vi "Globals.vi"(7 "action":T2, 8 "error in":errorcluster, 10 "Preliminary Settings":T1={"Nº of Scans (ns)"=3, "Pulse Frequency"=10000000.0} {"Pulse Frequency" min=1.0 format="%^#_6e"; "Nº of Scans (ns)" step=1}) -> (0 "error out":errorcluster, 2 "Preliminary Settings out":T1={"Nº of Scans (ns)"=3, "Pulse Frequency"=10000000.0} {"Pulse Frequency" min=1.0 format="%^#_6e"; "Nº of Scans (ns)" step=1})   [LabVIEW 2011]
uses:
  Globals.ctl
  Controls/Preliminary Settings.ctl
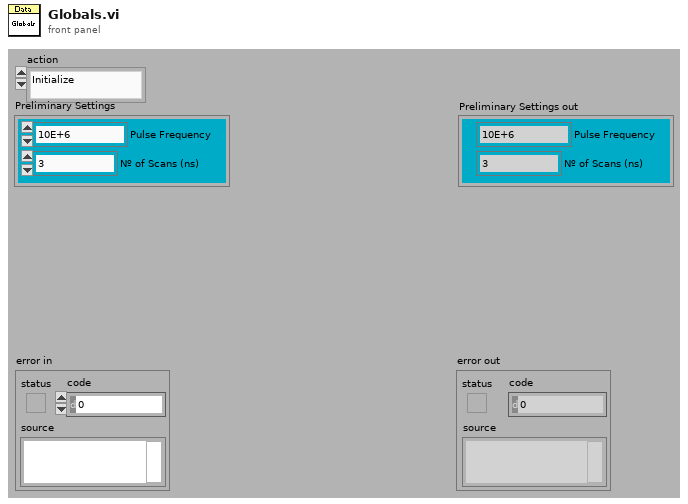
[diagram p1: front panel]
types:
  T1 = typedef "Preliminary Settings.ctl" = cluster{"Nº of Scans (ns)":u16, "Pulse Frequency":dbl}
  T2 = typedef "Globals.ctl" = enum16{"Initialize", "Set Preliminary Settings", "Get Preliminary Settings"}
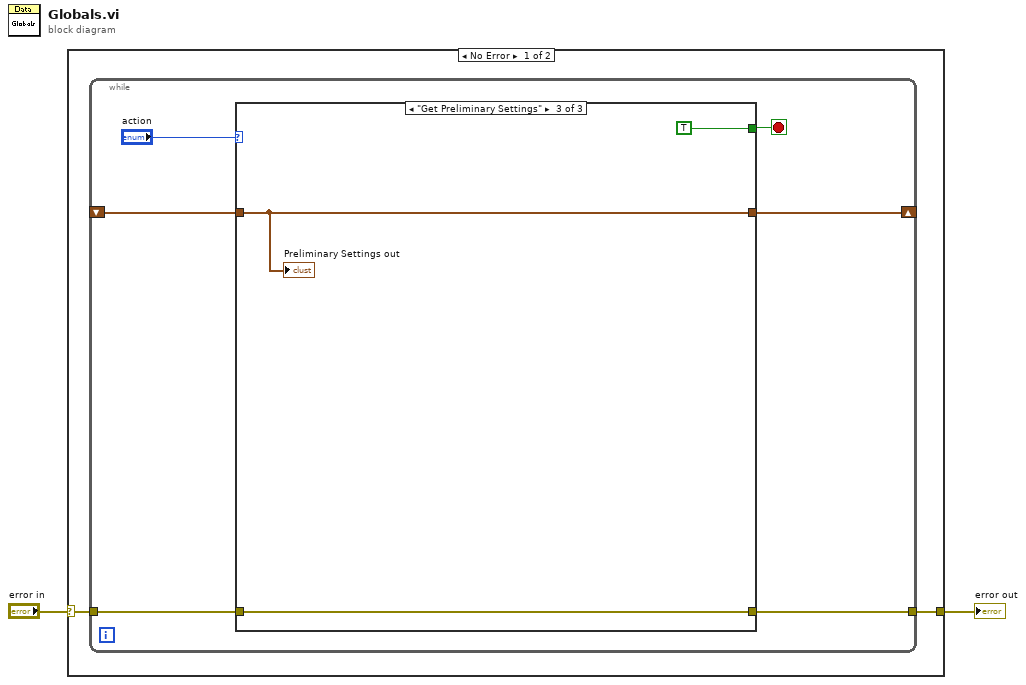
[diagram p0: block diagram]
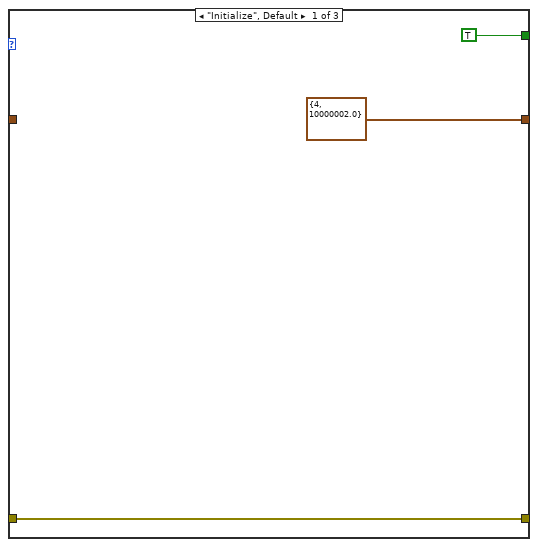
[diagram p2: hidden frame]
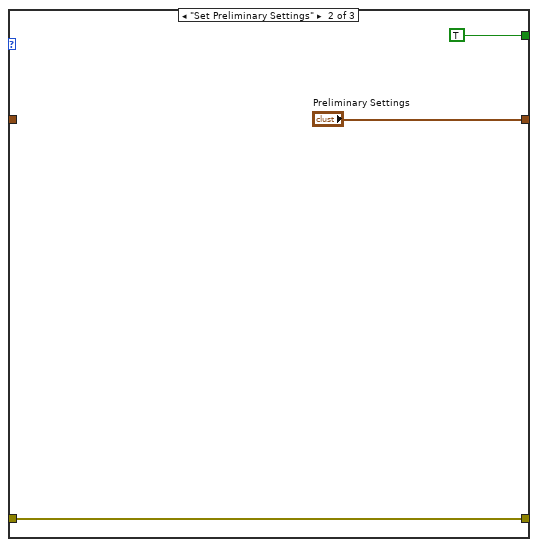
[diagram p3: hidden frame]
diagram:
  n1 = case shown="No Error" "error in" {
    selector: "error in" -> [w4 w20]
    tunnel: [w3 w20] -> w1
    frame No Error {
      n2 = while {
        tunnel: w4 -> [w9]
        tunnel: [w8] -> w3
        shift-right: [w6] -> _
        shift-left: _ -> [w5]
        stop <- w7 stop-if-true
        n3 = case shown="\"Get Preliminary Settings\"" "action" {
          tunnel: w9 -> [w12 w16 w19]
          tunnel: [w12 w16 w19] -> w8
          tunnel: [TRUE TRUE TRUE] -> w7
          tunnel: [T1 {"Nº of Scans (ns)"=4, "Pulse Frequency"=10000002.0} ("Preliminary Settings") "Preliminary Settings" w17] -> w6
          tunnel: w5 -> [_ _ w17]
          frame "Initialize", Default {
          }
          frame "Set Preliminary Settings" {
          }
          frame "Get Preliminary Settings" {
            "Preliminary Settings out" <- w17
          }
        }
      }
    }
    frame Error {
    }
  }
  "error out" <- w1
